vi "Encoder Velocity.vi"(6 "Initialize?":bool, 9 "Max sample interval (uS)":u32=62500, 10 "Encoder Count In":i64, 11 "Measurement Width (Counts)":i64=4) -> (1 "Enc Interval (uS)":u32, 2 "Enc Delta (Counts)":i64)   [LabVIEW 2016]
uses:
  <vilib>/rvi/Emulation/niFpgaCriticalErrorInLSC.vi
  <vilib>/rvi/Emulation/niFpgaEmulationReportErrorSimple.vi
  <vilib>/rvi/Emulation/niFpgaSctlEmulationGetInTimedLoop.vi
  <vilib>/rvi/Emulation/niFpgaGetClockAttributes.vi
panel:
  # "Inputs"
  # "Outputs"
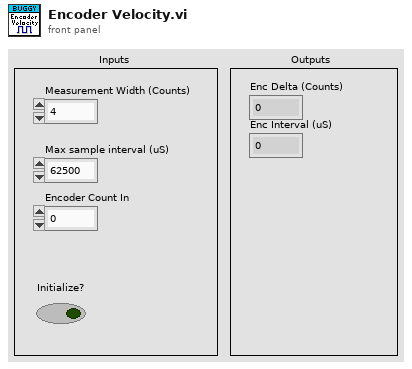
[diagram p1: front panel]
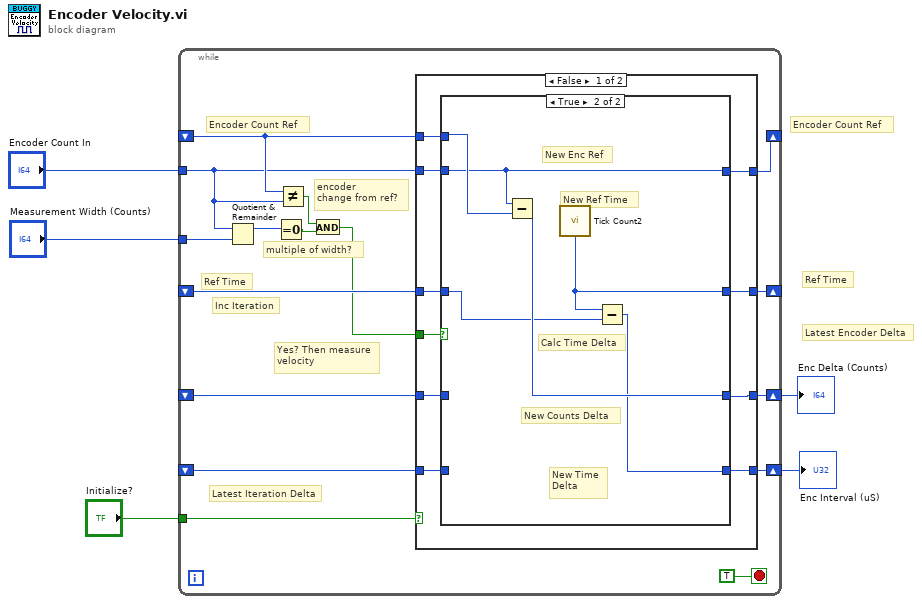
[diagram p0: block diagram]
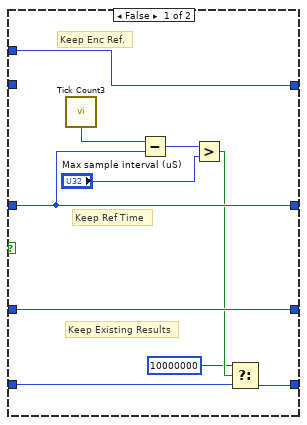
[diagram p2: hidden frame]
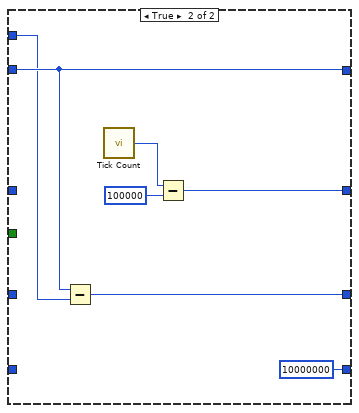
[diagram p3: hidden frame]
diagram:
  # "Latest Encoder Delta"
  # "Ref Time"
  # "Encoder Count Ref"
  n1 = while {
    shift-right: [w18] -> _
    shift-left: _ -> [w11]
    tunnel: "Initialize?" -> [w6]
    tunnel: "Measurement Width (Counts)" -> [w21]
    shift-right: [w19] -> _
    shift-left: _ -> [w8]
    tunnel: "Encoder Count In" -> [w10]
    shift-right: [w16] -> w2
    shift-left: _ -> [w14]
    shift-right: [w17] -> w1
    shift-left: _ -> [w13]
    stop <- TRUE stop-if-true
    # "Yes? Then measure\nvelocity"
    # "multiple of width?"
    # "encoder\nchange from ref?"
    # "Inc Iteration"
    # "Latest Iteration Delta"
    # "Encoder Count Ref"
    # "Ref Time"
    n2 = Quotient & Remainder(x=w10, y=w21) -> (x-y*floor(x/y)=w20:i64)  [unwired: 1 out]
    n3 = Equal To 0?(x=w20) -> (x = 0?=w12:bool)
    n4 = Not Equal?(x=w11, y=w10) -> (x != y?=w9:bool)
    n5 = And(x=w9, y=w12) -> (x .and. y?=w7:bool)
    n6 = case shown="False" w6 {
      tunnel: [w31 w51] -> w19
      tunnel: [w30 w50] -> w18
      tunnel: [w29 u32 10000000 ("t")] -> w17
      tunnel: [w28 w48] -> w16
      tunnel: w14 -> [w27 _]
      tunnel: w13 -> [w26 _]
      tunnel: w11 -> [w25 w49]
      tunnel: w10 -> [w24 w50]
      tunnel: w8 -> [w23 _]
      tunnel: w7 -> [w22 _]
      frame False {
        n7 = case shown="True" w22 {
          tunnel: [w38 w45] -> w31
          tunnel: [w41 w42] -> w30
          tunnel: [w34 w43] -> w29
          tunnel: [w40 w46] -> w28
          tunnel: w24 -> [_ w42]
          tunnel: w25 -> [w41 w47]
          tunnel: w27 -> [w40 _]
          tunnel: w26 -> [w32 _]
          tunnel: w23 -> [w38 w44]
          frame False {
            # "Keep Existing Results"
            # "Keep Ref Time"
            # "Keep Enc Ref."
            n8 = call "Tick Count3"() -> ("Tick Count(uSec)"=w39:u32)
            n9 = Subtract(x=w39, y=w38) -> (x-y=w36:u32)
            n10 = Greater?(x=w36, y="Max sample interval (uS)") -> (0:w35:bool)
            n11 = Select(t=u32 10000000, s=w35, f=w32) -> (s? t:f=w34:u32)
          }
          frame True {
            # "New Counts Delta"
            # "New Time\nDelta"
            # "Calc Time Delta"
            # "New Ref Time"
            # "New Enc Ref"
            n12 = Subtract(x=w42, y=w47) -> (x-y=w46:i64)
            n13 = call "Tick Count2"() -> ("Tick Count(uSec)"=w45:u32)
            n14 = Subtract(x=w45, y=w44) -> (x-y=w43:u32)
          }
        }
      }
      frame True {
        n15 = Subtract(x=w50, y=w49) -> (x-y=w48:i64)
        n16 = call "Tick Count"() -> ("Tick Count(uSec)"=w53:u32)
        n17 = Subtract(x=w53, y=u32 100000) -> (x-y=w51:u32)
      }
    }
  }
  "Enc Delta (Counts)" <- w2
  "Enc Interval (uS)" <- w1
